vi "Servo.vi"(4 "taskId":i32(ring) items=["TLibrary", "T01", "T02", "T03", "T04", "T05", "T06", "T07", "T08", "T09", "T10", "T11", "T12", "T13", "T14", "T15", "T16", "T17", "T18", "T19", "T20", "T21", "T22", "T23", "T24", "T25", "T26", "T27", "T28", "T29", "T30", "T31"], 6 "return immediately":bool, 8 "error in (no error)":errorcluster, 9 "on/off":i32(ring) items=["Off", "On"], 10 "axis name":string, 11 "controller":refnum<k24>) -> (0 "error out":errorcluster, 3 "controller out":refnum<k24>)   [LabVIEW 2020, in "Aerotech.lvlib"]
uses:
  Aerotech.lvlib
  C:/Users/HEP/Documents/GitHub/UCSB-Gantry-HEP/Drivers/Aerotech A3200/Bin/Aerotech.A3200.LabVIEW.dll
  UCSB-Gantry-HEP/Drivers/Aerotech A3200/Bin/Aerotech.A3200.LabVIEW.dll
  C:/Program Files (x86)/Aerotech/A3200/LabVIEW/2010/Bin/Aerotech.A3200.dll
  Program Files (x86)/Aerotech/A3200/LabVIEW/2010/Bin/Aerotech.A3200.dll
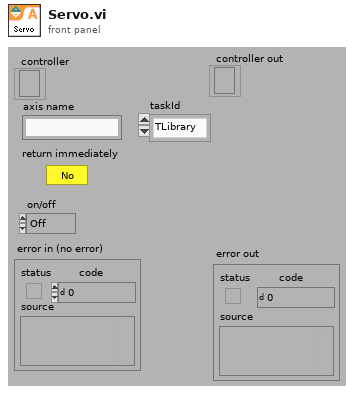
[diagram p1: front panel]
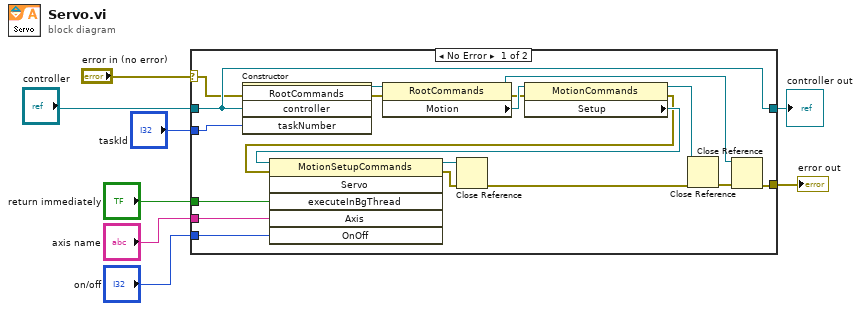
[diagram p0: block diagram]
diagram:
  n1 = case shown="No Error" "error in (no error)" {
    selector: "error in (no error)" -> [w12 w29]
    tunnel: [w20 w29] -> w7
    tunnel: "controller" -> [w13 w28]
    tunnel: "return immediately" -> [w25 _]
    tunnel: "axis name" -> [w24 _]
    tunnel: "on/off" -> [w23 _]
    tunnel: [w13 w28] -> w1
    tunnel: "taskId" -> [w9 _]
    frame No Error {
      n2 = constructor class="RootCommands"(error in=w12, "controller"=w13, "taskNumber"=w9) -> (reference out=w15:refnum<k24>, error out=w14:errorcluster)  [unwired: 2 in, 3 out]
      n3 = property class="RootCommands"(reference=w15, error in=w14) -> (reference out=w17:refnum<k24>, error out=w10:errorcluster, "Motion"=w11:refnum<k24>)
      n4 = property class="MotionCommands"(reference=w11, error in=w10) -> (reference out=w18:refnum<k24>, error out=w26:errorcluster, "Setup"=w27:refnum<k24>)
      n5 = invoke class="MotionSetupCommands" method="Servo"(reference=w27, error in=w26, "executeInBgThread"=w25, "Axis"=w24, "OnOff"=w23) -> (reference out=w21:refnum<k24>, error out=w22:errorcluster)  [unwired: 1 in, 4 out]
      n6 = Close Reference(reference=w21, error in (no error)=w22) -> (error out=w16:errorcluster)
      n7 = Close Reference(reference=w18, error in (no error)=w16) -> (error out=w19:errorcluster)
      n8 = Close Reference(reference=w17, error in (no error)=w19) -> (error out=w20:errorcluster)
    }
    frame Error {
    }
  }
  "error out" <- w7
  "controller out" <- w1
